vi "writeID.vi"(1 "ID":u32, 2 "ID Type":enum16{"Standard", "Extended"}(ring), 3 "Buffer Num":u8, 4 "SPI Config In":T1) -> (0 "SPI Config Out":T1)   [LabVIEW 2019]
uses:
  SPI/SPI Config.ctl
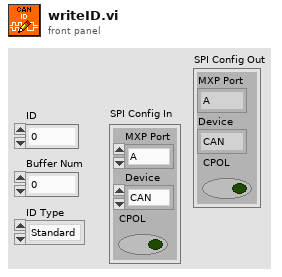
[diagram p1: front panel]
types:
  T1 = typedef "SPI Config.ctl" = cluster{"MXP Port":enum16{"A", "B"}, "Device":enum16{"CAN", "ENC", "IMU1", "IMU2"}, "CPOL":bool}
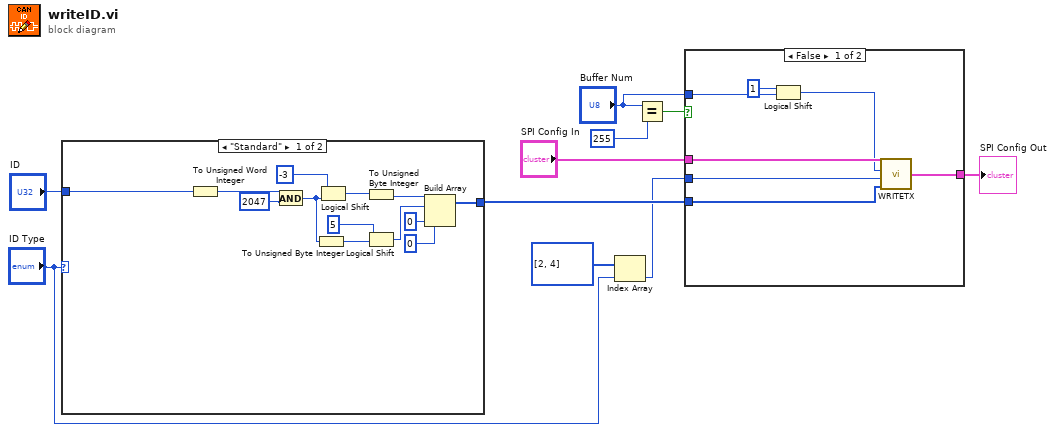
[diagram p0: block diagram]
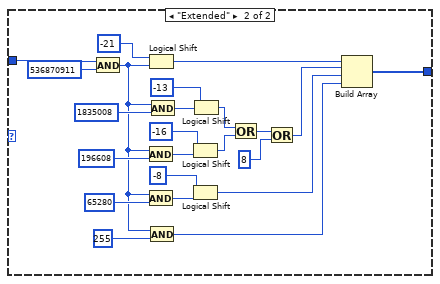
[diagram p2: hidden frame]
diagram:
  n1 = case shown="\"Standard\"" "ID Type" {
    tunnel: [w15 w24] -> w8
    tunnel: "ID" -> [w14 w46]
    frame "Standard" {
      n2 = To Unsigned Word Integer(number=w14) -> (unsigned 16bit integer=w13:u16)
      n3 = And(x=w13, y=u16 2047) -> (x .and. y?=w20:u16)
      n4 = To Unsigned Byte Integer(number=w20) -> (unsigned 8bit integer=w19:u8)
      n5 = Logical Shift(y=i16 -3, x=w20) -> (x << y=w21:u16)
      n6 = To Unsigned Byte Integer(number=w21) -> (unsigned 8bit integer=w17:u8)
      n7 = Logical Shift(y=i16 5, x=w19) -> (x << y=w16:u8)
      n8 = Build Array(w17, w16, u8 0 ("element"), u8 0 ("element")) -> (w15:u8[])
    }
    frame "Extended" {
      n9 = And(x=w46, y=u32 536870911) -> (x .and. y?=w27:u32)
      n10 = Logical Shift(y=i16 -21, x=w27) -> (x << y=w33:u32)
      n11 = And(x=w27, y=u32 196608) -> (x .and. y?=w39:u32)
      n12 = And(x=w27, y=u32 65280) -> (x .and. y?=w30:u32)
      n13 = And(x=w27, y=u32 255) -> (x .and. y?=w25:u32)
      n14 = And(x=w27, y=u32 1835008) -> (x .and. y?=w42:u32)
      n15 = Logical Shift(y=i16 -16, x=w39) -> (x << y=w37:u32)
      n16 = Logical Shift(y=i16 -8, x=w30) -> (x << y=w28:u32)
      n17 = Logical Shift(y=i16 -13, x=w42) -> (x << y=w36:u32)
      n18 = Or(x=w36, y=w37) -> (x .or. y?=w35:u32)
      n19 = Or(x=w35, y=u32 8) -> (x .or. y?=w32:u32)
      n20 = Build Array(w33, w32, w28, w25) -> (w24:u32[])
    }
  }
  n21 = Index Array(array=u8[] [2, 4], index="ID Type") -> (element=w1:u8)
  n22 = Equal?(x="Buffer Num", y=u8 255) -> (x = y?=w9:bool)
  n23 = case shown="False" w9 {
    tunnel: w8 -> [w50 _]
    tunnel: "Buffer Num" -> [w48 _]
    tunnel: "SPI Config In" -> [w52 w54]
    tunnel: [w51 w54] -> w4
    tunnel: w1 -> [w49 _]
    frame False {
      n24 = Logical Shift(y=i16 1, x=w48) -> (x << y=w47:u8)
      n25 = call "WRITETX.vi"("Data to Write"=w50, "Frames to Write"=w49, "Reg. Select"=w47, "SPI Config In"=w52) -> ("SPI Config Out"=w51:T1)
    }
    frame True {
    }
  }
  "SPI Config Out" <- w4
